vi "Live Image.vi"(8 "error in (no error)":errorcluster, 10 "Live.Data":T1, 11 "ImageHandler in":refnum<class "ImageHandler.lvclass">) -> (0 "error out":errorcluster, 3 "ImageHandler out":refnum<class "ImageHandler.lvclass">)   [LabVIEW 2022 SP3, in "ImageHandler.lvlib" / "ImageHandler.lvclass"]
uses:
  ImageHandler.lvclass
  ImageHandler.lvclass/ImageHandler.ctl
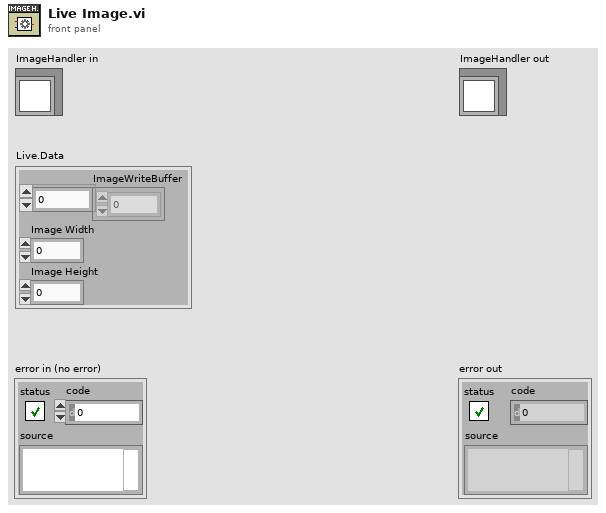
[diagram p1: front panel]
types:
  T1 = cluster{"ImageWriteBuffer":u16[], "Image Width":i32, "Image Height":i32}
  T2 = typedef "IMAQ Image.ctl" = refnum<image>
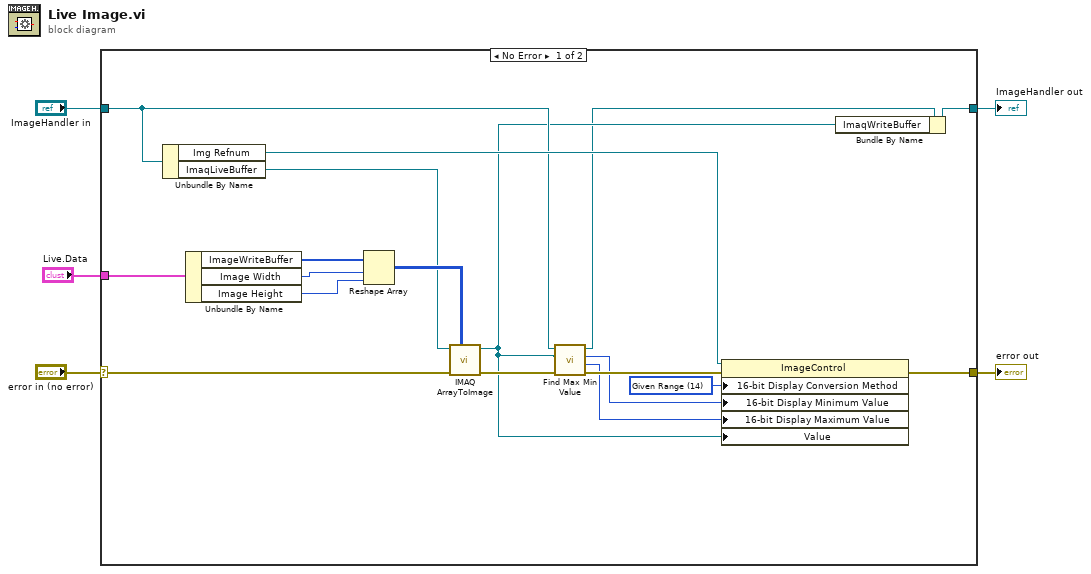
[diagram p0: block diagram]
diagram:
  n1 = case shown="No Error" "error in (no error)" {
    selector: "error in (no error)" -> [w17 w25]
    tunnel: [w16 w25] -> w4
    tunnel: [w13 w24] -> w2
    tunnel: "ImageHandler in" -> [w11 w24]
    tunnel: "Live.Data" -> [w15 _]
    frame No Error {
      w9 = u32 14 items=["Default"=10, "Most Significant Bits"=11, "Full Dynamic"=12, "Downshift"=13, "Given Range"=14, "90% Dynamic"=15, "Given Percent Range"=16] ("16-bit Display Mapping:Conversion Method")
      n2 = Unbundle By Name(w11) -> ("Img Refnum"=w14:refnum<vi>, "ImaqLiveBuffer"=w18:T2)
      n3 = Unbundle By Name(w15) -> ("ImageWriteBuffer"=w21:u16[], "Image Width"=w23:i32, "Image Height"=w22:i32)
      n4 = Reshape Array(w21, w23, w22) -> (w20:u16[][])
      n5 = call "IMAQ ArrayToImage"("Image Pixels (U16)"=w20, "error in (no error)"=w17, "Image"=w18) -> ("error out"=w19:errorcluster, "Image Out"=w10:T2)  [unwired: 7 in]
      n6 = call-dynamic "Find Max Min Value.vi"("error in (no error)"=w19, "ImageIn"=w10, "ImageHandler in"=w11) -> ("error out"=w12:errorcluster, "Maximal Value"=w7:i32, "Minimal Value"=w8:i32, "ImageHandler out"=w6:refnum<class "ImageHandler.lvclass">)  [unwired: 5 in]
      n7 = property class="ImageControl"(reference=w14, error in=w12, "16-bit Display Conversion Method"=w9, "16-bit Display Minimum Value"=w8, "16-bit Display Maximum Value"=w7, "Value"=w10) -> (error out=w16:errorcluster)  [unwired: 1 out]
      n8 = Bundle By Name(cluster=w6, "ImaqWriteBuffer"=w10) -> (w13:refnum<class "ImageHandler.lvclass">)
    }
    frame Error {
    }
  }
  "error out" <- w4
  "ImageHandler out" <- w2
